vi "Step End Action.vi"(8 "error in (no error)":errorcluster, 10 "Step":refnum<class "Step.lvclass">, 11 "Tester in":refnum<class "Tester.lvclass">) -> (0 "error out":errorcluster, 2 "Terminate":bool, 3 "Tester out":refnum<class "Tester.lvclass">)   [LabVIEW 2020, in "Tester.lvlib" / "Tester.lvclass"]
uses:
  Tester.lvclass
  Step/Step.lvclass
  <vilib>/Utility/error.llb/DialogType.ctl
  Results/Result.ctl
  Results/Results.lvclass
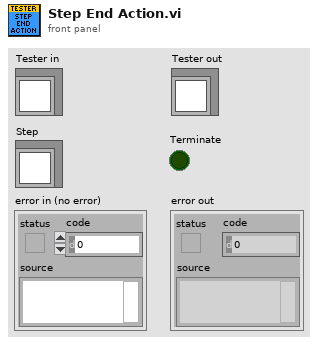
[diagram p1: front panel]
types:
  T1 = typedef "Tester.lvlib/Results.lvclass/Result.ctl" = enum16{"No Result", "Pass", "Fail", "Error", "Abort"}
  T2 = typedef "DialogType.ctl" = u16
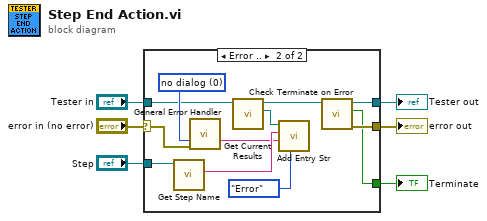
[diagram p0: block diagram]
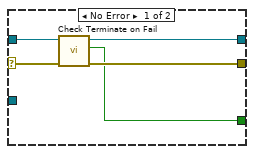
[diagram p2: hidden frame]
diagram:
  n1 = case shown="Error .." "error in (no error)" {
    selector: "error in (no error)" -> [w10 w23]
    tunnel: "Tester in" -> [w11 w20]
    tunnel: "Step" -> [_ w21]
    tunnel: [w9 w14] -> w3
    tunnel: [w8 w13] -> w2
    tunnel: [w7 w12] -> w1
    frame No Error {
      n2 = call "Check Terminate on Fail.vi"("error in (no error)"=w10, "Tester in"=w11) -> ("error out"=w8:errorcluster, "Terminate"=w7:bool, "Tester out"=w9:refnum<class "Tester.lvclass">)  [unwired: 7 in]
    }
    frame Error {
      w22 = T2 0 items=["no dialog", "OK message", "continue or stop message", "OK message + warnings", "continue/stop + warnings"] ("type of dialog (OK msg:1)")
      n3 = call-dynamic "Get Step Name.vi"("Step in"=w21) -> ("Step Name"=w18:string)  [unwired: 8 in, 2 out]
      n4 = call <vilib>:"General Error Handler.vi"("type of dialog (OK msg:1)"=w22, "error in (no error)"=w23) -> ("message"=w17:string)  [unwired: 9 in, 4 out]
      n5 = call "Get Current Results.vi"("Tester in"=w20) -> ("Current Results"=w19:refnum<class "Results.lvclass">, "Tester out"=w15:refnum<class "Tester.lvclass">)  [unwired: 8 in, 1 out]
      n6 = call "Add Entry Str.vi"("Result"=Result."Error", "Value Str"=w17, "Name"=w18, "Results in"=w19) -> ()  [unwired: 6 in, 2 out]
      n7 = call "Check Terminate on Error.vi"("Tester in"=w15) -> ("error out"=w13:errorcluster, "Stop on Error"=w12:bool, "Tester out"=w14:refnum<class "Tester.lvclass">)  [unwired: 8 in]
    }
  }
  "error out" <- w2
  "Tester out" <- w3
  "Terminate" <- w1
